vi "Update.vi"(8 "error in (no error)":errorcluster, 11 "MainMenu in":refnum<class "MainMenu.lvclass">) -> (0 "error out":errorcluster, 3 "MainMenu out":refnum<class "MainMenu.lvclass">)   [LabVIEW 2019, in "RT_Game.lvlib" / "MainMenu.lvclass"]
uses:
  MainMenu.lvclass
  C:/Users/FreshBob/Dropbox/VIs/myRIO_GameConsole/RT/RT_Game/Game/Game.lvclass
  Game/Game.lvclass/Game.ctl
  MainMenu.lvclass/MainMenu.ctl
  Game/Read Sprites.vi
  Game/Write Sprites.vi
  RT_Sprite/RT_Sprite.lvclass
  C:/Users/FreshBob/Dropbox/VIs/myRIO_GameConsole/RT/RT_Game/GameObject/GameObject.lvclass
  Menu/Menu.lvclass
  GameObject/GameObject.lvclass
  Game/Game.lvclass
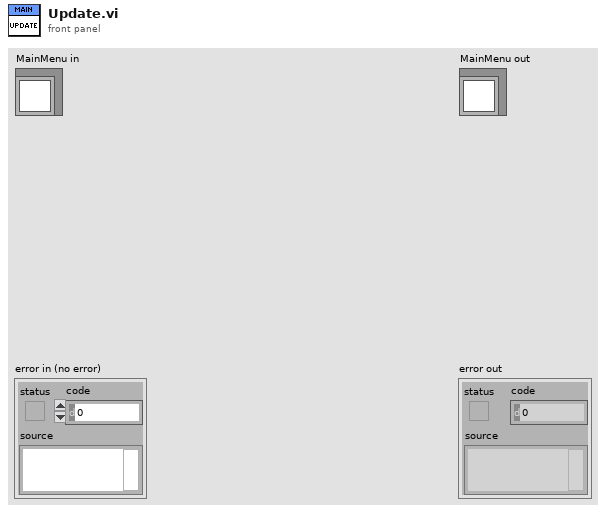
[diagram p1: front panel]
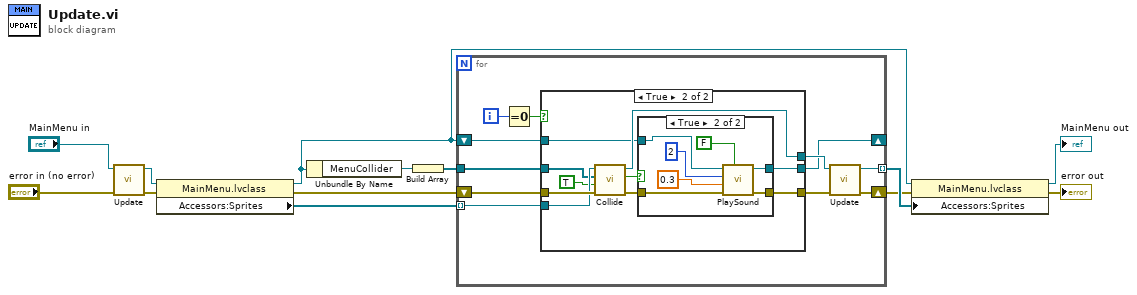
[diagram p0: block diagram]
diagram:
  n1 = call-parent "Update.vi"("error in (no error)"="error in (no error)", "Menu in"="MainMenu in") -> ("error out"=w13:errorcluster, "Menu out"=w10:refnum<class "MainMenu.lvclass">)  [unwired: 8 in]
  n2 = property class="MainMenu.lvclass"(reference=w10, error in=w13) -> (reference out=w1:refnum<class "MainMenu.lvclass">, error out=w6:errorcluster, "Accessors:Sprites"=w4:refnum<class "RT_Sprite.lvclass">[])
  n3 = Unbundle By Name(w1) -> ("MenuCollider"=w3:refnum<class "GameObject.lvclass">)
  n4 = Build Array(w3) -> (w2:refnum<class "GameObject.lvclass">[])
  n5 = for {
    tunnel: w4 -> [w19] mode=indexing
    tunnel: [w22] -> w7 mode=indexing
    shift-right: [w23] -> w5
    shift-left: w6 -> [w24]
    tunnel: w2 -> [w18]
    shift-right: [w14] -> _
    shift-left: w1 -> [w15]
    i -> [w17]
    n6 = Equal To 0?(x=w17) -> (x = 0?=w16:bool)
    n7 = case shown="True" w16 {
      tunnel: w24 -> [w26 w37]
      tunnel: [w26 w31] -> w21
      tunnel: [w27 w35] -> w20
      tunnel: w19 -> [w27 w34]
      tunnel: w18 -> [_ w33]
      tunnel: [w25 w29] -> w14
      tunnel: w15 -> [w25 w30]
      frame False {
      }
      frame True {
        n8 = call "Collide.vi"("error in (no error)"=w37, "CollideAll?"=TRUE, "Colliders"=w33, "Object in"=w34) -> ("error out"=w36:errorcluster, "collided"=w28:bool, "Object out"=w35:refnum<class "RT_Sprite.lvclass">)  [unwired: 5 in]
        n9 = case shown="True" w28 {
          tunnel: w36 -> [w39 w46]
          tunnel: [w39 w45] -> w31
          tunnel: w30 -> [w38 w44]
          tunnel: [w38 w43] -> w29
          frame False {
          }
          frame True {
            n10 = call "PlaySound.vi"("Overwrite? (T)"=FALSE, "error in (no error)"=w46, "Volume(0..1)"=0.3, "Index"=i16 2, "Game in"=w44) -> ("error out"=w45:errorcluster, "Game out"=w43:refnum<class "MainMenu.lvclass">)  [unwired: 5 in]
          }
        }
      }
    }
    n11 = call-dynamic "Update.vi"("error in (no error)"=w21, "GameObject in"=w20) -> ("error out"=w23:errorcluster, "GameObject out"=w22:refnum<class "RT_Sprite.lvclass">)  [unwired: 8 in]
  }
  n12 = property class="MainMenu.lvclass"(reference=w1, error in=w5, "Accessors:Sprites"=w7) -> (reference out=→"MainMenu out":refnum<class "MainMenu.lvclass">, error out=→"error out":errorcluster)
